vi "Output Power--SubVI.vi"(4 "Instance(1)":i32=1, 8 "error in (no error)":errorcluster, 11 "Watlow F4T In":refnum<class "Watlow F4T.lvclass">) -> (0 "error out":errorcluster, 2 "Output (+/-100%)":dbl, 3 "Watlow F4T out":refnum<class "Watlow F4T.lvclass">)   [LabVIEW 2024, in "Watlow F4T.lvclass"]
uses:
  Watlow F4T.lvclass
  Private/Controls/Standard Bus Commands--Enum.ctl
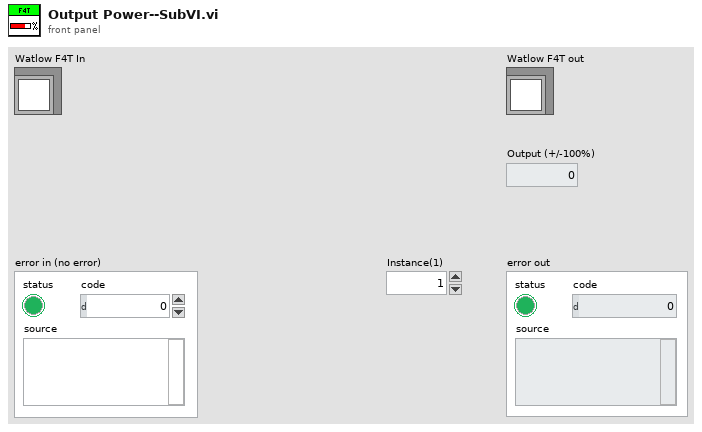
[diagram p1: front panel]
types:
  T1 = typedef "Watlow F4T.lvclass/Standard Bus Commands--Enum.ctl" = enum16{"Remote Setpoint", "Remote Mode", "Temp Feedback", "Target Setpoint", "Current Setpoint", "Setpoint Lower Limit", "Setpoint Upper Limit", "Ramp Rate Y", "Ramp Rate X", "Ramp Rate Action", "Temp Control State", "Temp Control Mode", "Power", "Heat Power", "Cool Power"}
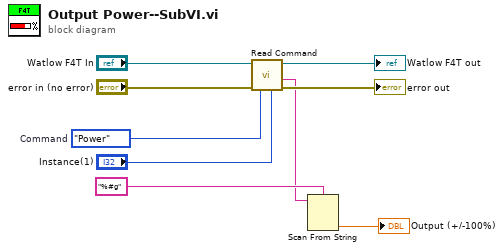
[diagram p0: block diagram]
diagram:
  w5 = Standard_Bus_Commands--Enum."Power"  # Command
  n1 = call "Read Command.vi"("Instance"="Instance(1)", "Commands"=w5, "error in (no error)"="error in (no error)", "Watlow F4T In"="Watlow F4T In") -> ("error out"=→"error out":errorcluster, "Value Out"=w2:string, "Watlow F4T out"=→"Watlow F4T out":refnum<class "Watlow F4T.lvclass">)  [unwired: 5 in]
  n2 = Scan From String(format string="%#g", input string=w2) -> (output 1=→"Output (+/-100%)":dbl)  [unwired: 3 in, 3 out]
